vi "Untitled 4.vi"() -> ()   [LabVIEW 2017]
uses:
  <vilib>/userdefined/High Color/IMAQdx.ctl
panel:
  in  "Rectangle":T1 {"Rotation" min=-90.0 max=90.0 step=1.0 format="%.2f"; "Left" scale=0.0..1024.0; "Right" scale=0.0..1024.0}
  out "Editted HSL Image 2":T2(plugin-control)
  out "Editted L Image 2":T2(plugin-control)
  out "Editted S Image 2":T2(plugin-control)
  out "Editted H Image 2":T2(plugin-control)
  out "Real-Image":T2(plugin-control)
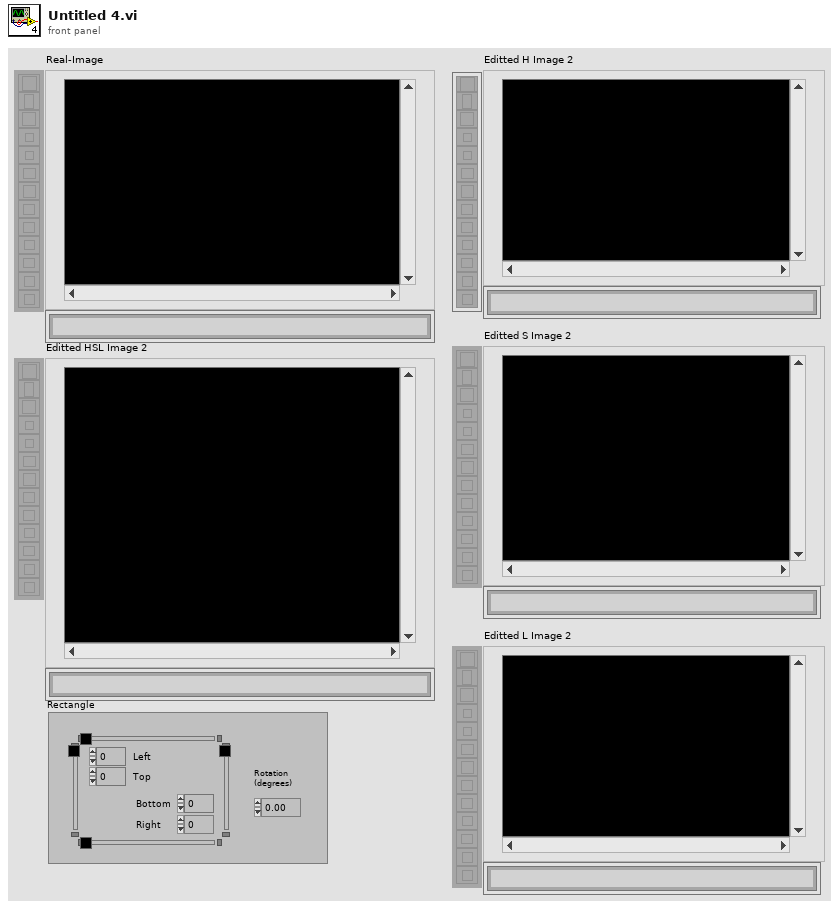
[diagram p1: front panel]
types:
  T1 = typedef "IMAQ Rectangle" = cluster{"Left":i32, "Top":i32, "Right":i32, "Bottom":i32, "Rotation":dbl}
  T2 = typedef "IMAQ Image.ctl" = refnum<image>
  T3 = typedef "Image Type" = u32
  T4 = typedef "IMAQdx.ctl" = refnum<k21>
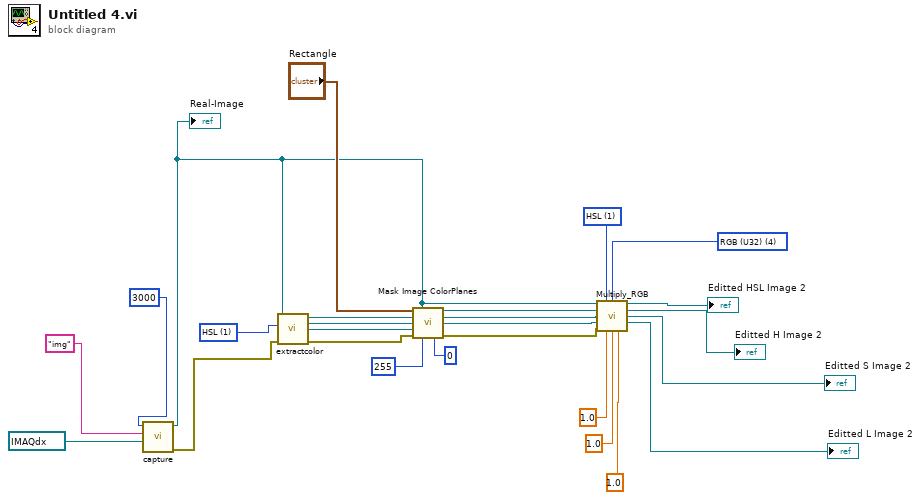
[diagram p0: block diagram]
diagram:
  w23 = u16 1 items=["RGB", "HSL", "HSV", "HSI"] ("Color Mode")
  w21 = T3 4 items=["Grayscale (U8)", "Grayscale (I16)", "Grayscale (SGL)", "Complex (CSG)", "RGB (U32)", "HSL (U32)", "RGB (U64)", "Grayscale (U16)"] ("ImageOutput Type")
  w22 = u16 1 items=["RGB", "HSL", "HSV", "HSI"] ("Color Mode")
  n1 = call "capture.vi"("Session In"=T4 "cam3", "Image Name"="img", "Timeout (ms)"=3000) -> ("error out 4"=w14:errorcluster, "Image"=w4:T2)  [unwired: 7 in]
  "Real-Image" <- w4
  n2 = call "extractcolor.vi"("error in (no error)"=w14, "Color Mode"=w23, "Image Src"=w4) -> ("error out Extract"=w6:errorcluster, "Blue or Luma or Val or Inten Plane out"=w7:T2, "Green or Sat Plane out"=w8:T2, "Red or Hue Plane out"=w9:T2)  [unwired: 5 in]
  n3 = call "Mask Image ColorPlanes.vi"("Rectangle"="Rectangle", "Image Model"=w4, "Image R/H"=w9, "Image G/S"=w8, "Image B/L"=w7, "error in (no error)"=w6, "Filling Value (255)"=255, "Background Value (0)"=0) -> ("R/HMasked_Image"=w5:T2, "G/SMasked_Image"=w3:T2, "B/LMasked_Image"=w2:T2, "error out"=w1:errorcluster)  [unwired: 4 in]
  n4 = call "Multiply_RGB.vi"("Image Src"=w4, "Color Mode"=w22, "ImageOutput Type"=w21, "R/Hue Image Src"=w5, "G/Sat Image Src"=w3, "B/Luma/Val Image Src"=w2, "error in (no error)"=w1, "R/Hue Constant"=1.0, "G/Sat Constant"=1.0, "B/Luma/Val Constant"=1.0) -> ("Image Dst Out"=→"Editted HSL Image 2":T2, "R/Hue Out"=→"Editted H Image 2":T2, "G/Sat Out"=→"Editted S Image 2":T2, "B/Luma/Val Out"=→"Editted L Image 2":T2)  [unwired: 1 in, 1 out]
